vi "MB Registers Manager.vi"(5 "Function":enum16{"Init", "Read", "Write", "Read All"}(ring), 6 "Bits In":bool[](array[boolean]), 7 "Table":T1(ring), 8 "error in (no error)":errorcluster, 9 "Words In":u16[](array[numeric]), 10 "Length":u16, 11 "Start Address":u16) -> (0 "error out":errorcluster, 1 "Words out":u16[](array[numeric]), 4 "Bits out":bool[](array[boolean]))   [LabVIEW 2023, in "Voegtlin_NI_SMART_Modbus_Drivers.lvlib"]
uses:
  Voegtlin_NI_SMART_Modbus_Drivers.lvlib
panel:
  # "VI Name: MB Registers Manager.vi\nPurpose: Read/Write Local Slave Registers."
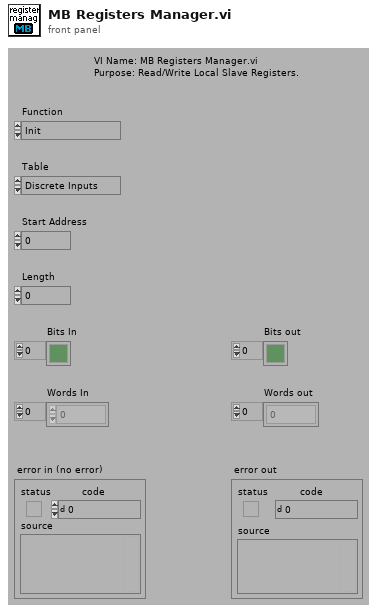
[diagram p1: front panel]
types:
  T1 = enum16{"Discrete Inputs", "Coils", "Input Registers", "Holding Registers"}
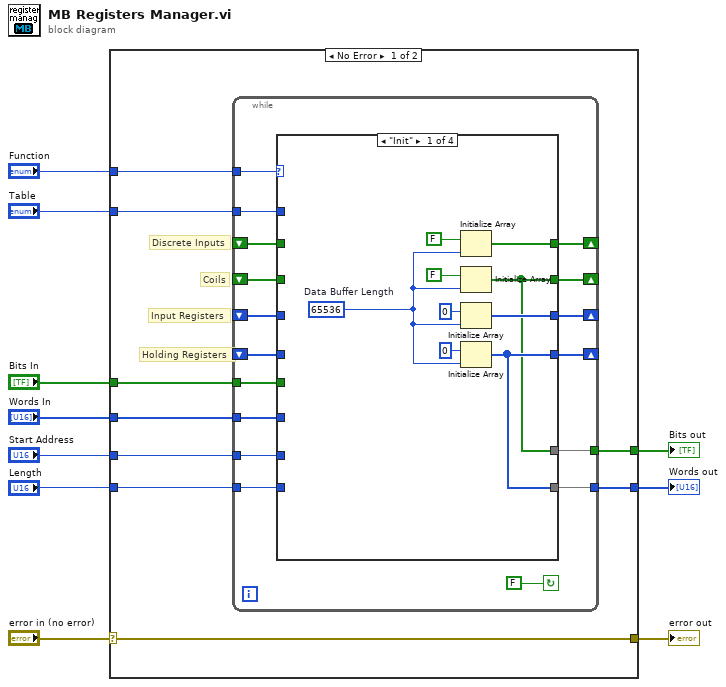
[diagram p0: block diagram]
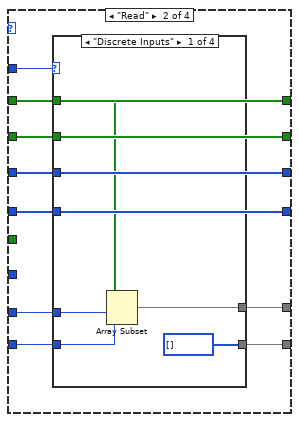
[diagram p2: hidden frame]
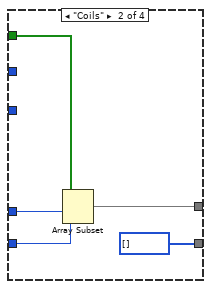
[diagram p3: hidden frame]
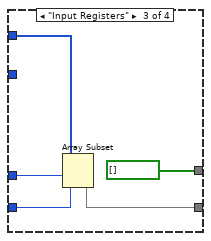
[diagram p4: hidden frame]
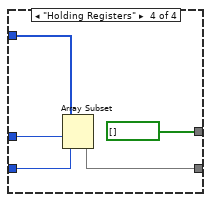
[diagram p5: hidden frame]
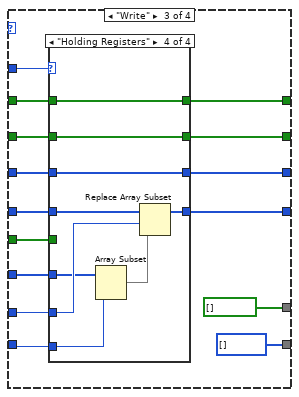
[diagram p6: hidden frame]
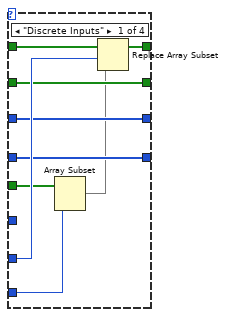
[diagram p7: hidden frame]
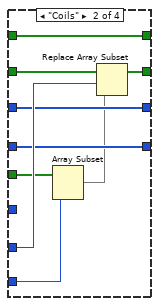
[diagram p8: hidden frame]
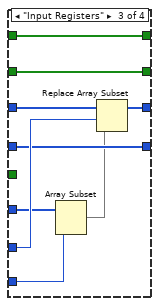
[diagram p9: hidden frame]
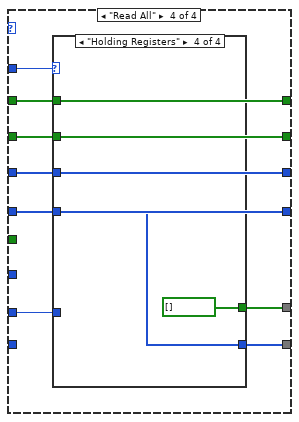
[diagram p10: hidden frame]
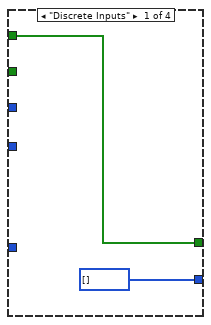
[diagram p11: hidden frame]
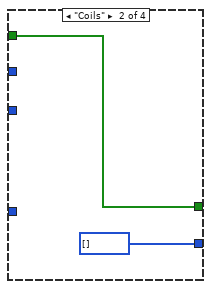
[diagram p12: hidden frame]
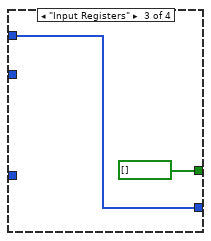
[diagram p13: hidden frame]
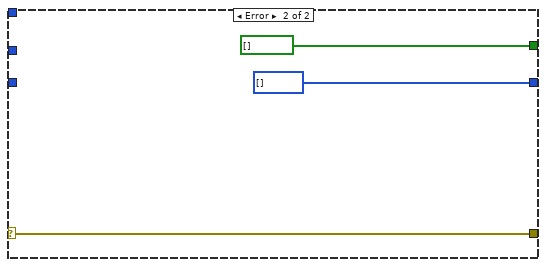
[diagram p14: hidden frame]
diagram:
  n1 = case shown="No Error" "error in (no error)" {
    selector: "error in (no error)" -> [w19 w144]
    tunnel: [w19 w144] -> w9
    tunnel: [w18 bool[] [] ("words out")] -> w8
    tunnel: [w17 u16[] [] ("words out")] -> w7
    tunnel: "Length" -> [w16 _]
    tunnel: "Start Address" -> [w15 _]
    tunnel: "Bits In" -> [w14 _]
    tunnel: "Words In" -> [w13 _]
    tunnel: "Function" -> [w12 _]
    tunnel: "Table" -> [w11 _]
    frame No Error {
      # "Holding Registers"
      # "Input Registers"
      # "Coils"
      # "Discrete Inputs"
      n2 = while {
        shift-right: [w35] -> _
        shift-left: _ -> [w33]
        shift-right: [w34] -> _
        shift-left: _ -> [w32]
        tunnel: [w31] -> w18
        tunnel: [w30] -> w17
        tunnel: w16 -> [w29]
        tunnel: w15 -> [w28]
        tunnel: w14 -> [w27]
        tunnel: w13 -> [w26]
        tunnel: w12 -> [w25]
        shift-right: [w23] -> _
        shift-left: _ -> [w20]
        shift-right: [w24] -> _
        shift-left: _ -> [w21]
        tunnel: w11 -> [w22]
        stop <- FALSE continue-if-true
        n3 = case shown="\"Init\"" w25 {
          tunnel: [w43 w46 w81 w126] -> w35
          tunnel: [w42 w50 w83 w130] -> w34
          tunnel: w33 -> [_ w46 w84 w126]
          tunnel: w28 -> [_ w53 w88 w132]
          tunnel: w26 -> [_ _ w76 _]
          tunnel: [w43 w49 u16[] [] ("Words In") w129] -> w30
          tunnel: w32 -> [_ w50 w87 w130]
          tunnel: [w37 w51 bool[] [] ("Bits In") w131] -> w31
          tunnel: w29 -> [_ w52 w75 _]
          tunnel: w27 -> [_ _ w82 _]
          tunnel: [w37 w48 w79 w128] -> w24
          tunnel: [w38 w47 w80 w127] -> w23
          tunnel: w22 -> [_ w54 w89 w133]
          tunnel: w21 -> [_ w48 w86 w128]
          tunnel: w20 -> [_ w47 w85 w127]
          frame "Init" {
            w39 = 65536  # Data Buffer Length
            n4 = Initialize Array(FALSE, w39) -> (w42:bool[])
            n5 = Initialize Array(FALSE, w39) -> (w37:bool[])
            n6 = Initialize Array(u16 0, w39) -> (w38:u16[])
            n7 = Initialize Array(u16 0, w39) -> (w43:u16[])
          }
          frame "Read" {
            n8 = case shown="\"Discrete Inputs\"" w54 {
              tunnel: w50 -> [w57 _ _ _]
              tunnel: w53 -> [w59 w64 w69 w74]
              tunnel: w52 -> [w58 w63 w68 w73]
              tunnel: [w56 w62 bool[] [] ("Bits In") bool[] [] ("Bits In")] -> w51
              tunnel: [u16[] [] ("Words In") u16[] [] ("Words In") w65 w71] -> w49
              tunnel: w48 -> [_ w60 _ _]
              tunnel: w47 -> [_ _ w67 _]
              tunnel: w46 -> [_ _ _ w70]
              frame "Discrete Inputs" {
                n9 = Array Subset(array=w57, index=w59, length=w58) -> (w56:bool[])
              }
              frame "Coils" {
                n10 = Array Subset(array=w60, index=w64, length=w63) -> (w62:bool[])
              }
              frame "Input Registers" {
                n11 = Array Subset(array=w67, index=w69, length=w68) -> (w65:u16[])
              }
              frame "Holding Registers" {
                n12 = Array Subset(array=w70, index=w74, length=w73) -> (w71:u16[])
              }
            }
          }
          frame "Write" {
            n13 = case shown="\"Holding Registers\"" w89 {
              tunnel: w87 -> [w98 w102 w114 w124]
              tunnel: w88 -> [w96 w107 w116 w125]
              tunnel: w86 -> [w93 w104 w111 w123]
              tunnel: w85 -> [w94 w105 w113 w120]
              tunnel: w84 -> [w95 w106 w115 w122]
              tunnel: [w97 w102 w114 w124] -> w83
              tunnel: w82 -> [w92 w101 _ _]
              tunnel: [w95 w106 w115 w121] -> w81
              tunnel: [w94 w105 w112 w120] -> w80
              tunnel: [w93 w103 w111 w123] -> w79
              tunnel: w76 -> [_ _ w110 w119]
              tunnel: w75 -> [w90 w99 w108 w117]
              frame "Discrete Inputs" {
                n14 = Array Subset(array=w92, length=w90) -> (w91:bool[])  [unwired: 1 in]
                n15 = Replace Array Subset(array=w98, new element=w91, index=w96) -> (w97:bool[])
              }
              frame "Coils" {
                n16 = Array Subset(array=w101, length=w99) -> (w100:bool[])  [unwired: 1 in]
                n17 = Replace Array Subset(array=w104, new element=w100, index=w107) -> (w103:bool[])
              }
              frame "Input Registers" {
                n18 = Array Subset(array=w110, length=w108) -> (w109:u16[])  [unwired: 1 in]
                n19 = Replace Array Subset(array=w113, new element=w109, index=w116) -> (w112:u16[])
              }
              frame "Holding Registers" {
                n20 = Array Subset(array=w119, length=w117) -> (w118:u16[])  [unwired: 1 in]
                n21 = Replace Array Subset(array=w122, new element=w118, index=w125) -> (w121:u16[])
              }
            }
          }
          frame "Read All" {
            n22 = case shown="\"Holding Registers\"" w133 {
              tunnel: w130 -> [w134 _ _ _]
              tunnel: w132 -> [_ _ _ _]
              tunnel: [w134 w136 bool[] [] bool[] []] -> w131
              tunnel: [u16[] [] ("Words In") u16[] [] ("Words In") w139 w140] -> w129
              tunnel: w128 -> [_ w136 _ _]
              tunnel: w127 -> [_ _ w139 _]
              tunnel: w126 -> [_ _ _ w140]
              frame "Discrete Inputs" {
              }
              frame "Coils" {
              }
              frame "Input Registers" {
              }
              frame "Holding Registers" {
              }
            }
          }
        }
      }
    }
    frame Error {
    }
  }
  "error out" <- w9
  "Bits out" <- w8
  "Words out" <- w7
